vi "Measurement Logic.vi"(8 "error in":errorcluster, 11 "Measurement Configuration":T2) -> (0 "error out":errorcluster, 3 "Measurement Results":T1)   [LabVIEW 2020, in "MeasurementTemplate_server.lvlib"]
uses:
  MeasurementTemplate_server.lvlib
  Measurement Configuration.ctl
  Measurement Results.ctl
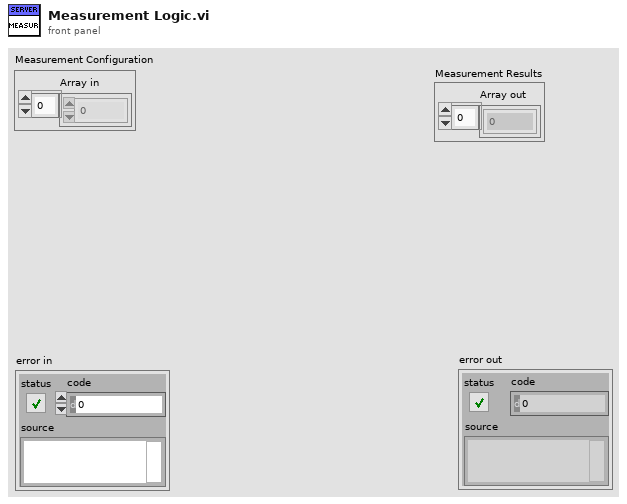
[diagram p1: front panel]
types:
  T1 = typedef "MeasurementTemplate_server.lvlib/Measurement Results.ctl" = cluster{"Array out":dbl[]}
  T2 = typedef "MeasurementTemplate_server.lvlib/Measurement Configuration.ctl" = cluster{"Array in":dbl[]}
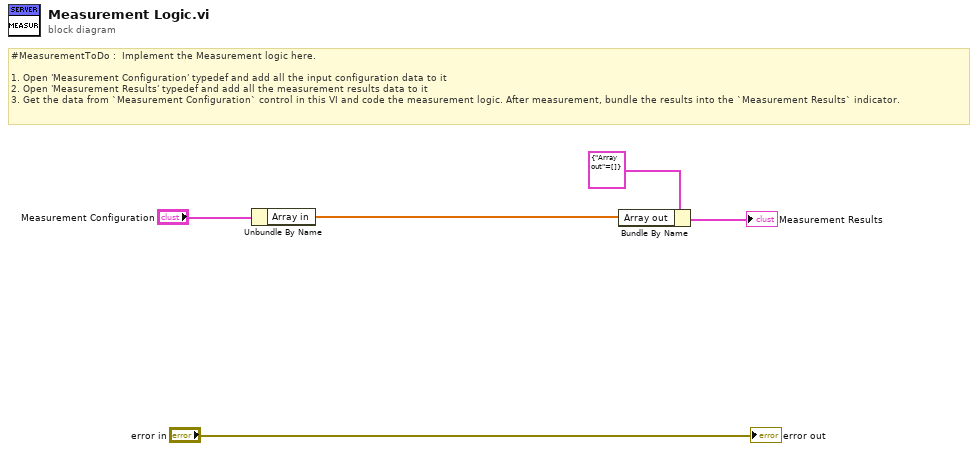
[diagram p0: block diagram]
diagram:
  # "#MeasurementToDo :  Implement the Measurement logic here.\n\n1. Open 'Measurement Configuration' typedef and add all the input configuration data to it\n2. Open 'Measurement Results' typedef and add all the measurement results data to it\n3. Get the data from `Measurement Configuration` control in this VI and code the measurement logic. After measurement, bundle the results into the `Measurement Results` indicator."
  n1 = Unbundle By Name("Measurement Configuration") -> ("Array in"=w2:dbl[])
  n2 = Bundle By Name(cluster=T1 {"Array out"=[]} ("Measurement Results"), "Array out"=w2) -> (→"Measurement Results":T1)
  "error out" <- "error in"
